vi "count_r3.vi"() -> ()   [LabVIEW 2015]
uses:
  <vilib>/myRIO/Instrument Drivers/Onboard IO/PWM/typedefs/PWM Reference.ctl
  <vilib>/myRIO/Common/Instrument Driver Framework/Utilities/typedefs/myRIO Generic Hardware Reference.ctl
  <vilib>/myRIO/Common/Instrument Driver Framework/Utilities/typedefs/Hardware Version Enum.ctl
  <vilib>/myRIO/Common/Instrument Driver Framework/Utilities/typedefs/myRIO v1.0 Reference.ctl
  <vilib>/myRIO/Common/Instrument Driver Framework/Utilities/typedefs/Generic FPGA Reference.ctl
  <vilib>/myRIO/Common/Instrument Driver Framework/myRIO v1.0/PWM/typedefs/PWM Channels Enum.ctl
  <vilib>/myRIO/Instrument Drivers/Onboard IO/PWM/typedefs/PWM Configuration.ctl
  <vilib>/userdefined/High Color/nirio_resource_hc.ctl
  <vilib>/myRIO/Common/Instrument Driver Framework/myRIO v1.0/PWM/vis/myRIO v1.1 Open PWM.vi
  <vilib>/myRIO/Common/Instrument Driver Framework/Utilities/vis/Validate Channels.vi
  <vilib>/myRIO/Common/Instrument Driver Framework/myRIO v1.0/PWM/vis/myRIO v1.0 Reserve PWM.vi
  <vilib>/myRIO/Instrument Drivers/Onboard IO/PWM/vis/Set Duty Cycle and Frequency.vi
  <vilib>/myRIO/Common/Instrument Driver Framework/myRIO v1.0/PWM/vis/myRIO v1.0 Build MUX Configuration PWM.vi
  <vilib>/myRIO/Common/Instrument Driver Framework/myRIO v1.0/Resource Manager/vis/myRIO v1.0 Reserve Channel List.vi
  <vilib>/myRIO/Common/Instrument Driver Framework/myRIO v1.0/Resource Manager/vis/myRIO v1.0 Create Configuration List.vi
  <vilib>/myRIO/Common/Instrument Driver Framework/myRIO v1.0/Resource Manager/vis/myRIO v1.0 Reserve Channel.vi
  <vilib>/myRIO/Common/Instrument Driver Framework/myRIO v1.0/Resource Manager/vis/myRIO v1.0 Unreserve Channel.vi
  <vilib>/myRIO/Common/Instrument Driver Framework/myRIO v1.0/Resource Manager/vis/myRIO v1.0 Build Mutex Name.vi
  <vilib>/FPGAPlugInAG/myRIO-1900/niLvFpga_Open_myRIO-1900.vi
  <vilib>/rvi/interface/common/dynamic/niFpgaDynamicAddResources.vi
  <vilib>/myRIO/Common/Instrument Driver Framework/Utilities/vis/FPGA Ref Manager.vi
  <vilib>/Utility/error.llb/Error Cluster From Error Code.vi
  <vilib>/myRIO/Common/Instrument Driver Framework/Utilities/vis/Ref Counter.vi
  <vilib>/rvi/errors/niLvFpgaAdjustHostInterfaceError.vi
  <vilib>/Utility/VariantDataType/GetNumericInfo.vi
  <vilib>/myRIO/Common/Instrument Driver Framework/myRIO v1.0/myRIO v1.1 Open.vi
  <vilib>/myRIO/Common/Instrument Driver Framework/Utilities/vis/IO Manager.vi
  <vilib>/myRIO/Common/Instrument Driver Framework/Utilities/vis/Configuration Manager.vi
  <vilib>/myRIO/Common/Instrument Driver Framework/myRIO v1.0/Resource Manager/vis/myRIO v1.0 Configure IO.vi
  <vilib>/myRIO/Common/Instrument Driver Framework/myRIO v1.0/myRIO v1.0 Close.vi
  <vilib>/myRIO/Common/Instrument Driver Framework/myRIO v1.0/PWM/vis/myRIO v1.0 Write PWM.vi
  <vilib>/rvi/interface/nirviOpenFPGA/nirviOpenFPGA.xnode
  FPGA Bitfiles/NavigationProjec_FPGATarget2_FPGAMainNavigati_PWPHW8gwDxI.lvbitx
  <vilib>/rvi/interface/nirviReadWriteControl/nirviReadWriteControl.xnode
  <vilib>/myRIO/Instrument Drivers/Onboard IO/PWM/vis/myRIO PWM Open.xnode
  <vilib>/myRIO/Instrument Drivers/Onboard IO/PWM/PWM.lvlib
  <vilib>/myRIO/Instrument Drivers/Utilities/Utilities.lvlib
  NiFpgaLv.dll
  <vilib>/rvi/interface/Simulation/niFpgaSimulationCallBeginRW.vi
panel:
  in  "graph?":bool
  out "Tick Count(mSec)":u32
  out "reset x y":dbl
  out "XY Graph":cluster{dbl[], dbl[]}(graph)
  out "x traveled":dbl
  out "y traveled":dbl
  out "avg 123":dbl
  out "avg 456":dbl
  out "psi dot":dbl
  out "distance traveled":dbl
  out "y dot":dbl
  out "x dot":dbl
  out "x position":dbl
  out "y position":dbl
  out "X Pos Lin Estimate":dbl
  out "Delta Lin Distance (ft)":dbl
  out "X Position Estimate":dbl
  out "Delta Distance (ft)":dbl
  in  "start y":dbl=3.0
  in  "start x":dbl=1.0
  out "Delta Encoder Array":u32[](array[numeric])
  out "Current Encoder Array":u32[](array[numeric])
  out "Initial Encoder Array":u32[](array[numeric])
  in  "Encoder Reset":bool
  in  "master motor on switch":bool
  out "L Min Linear Velocity (ft/s) 2":dbl
  out "R Min Linear Velocity (ft/s)  2":dbl
  in  "Goal Y":dbl=3.0 format="%#_13g"
  in  "Goal X":dbl=20.0 format="%#_13g"
  out "x+y":dbl
  out "SYS.SELECTA":u8 format="%08b"
  out "ENC.B_c.CNTR":i32
  out "ENC.B_b.CNTR":i32
  out "ENC.B_a.CNTR":i32
  out "ENC.A_c.CNTR":i32
  out "ENC.A_b.CNTR":i32
  out "ENC.A_a.CNTR":i32
  out "Boolean":bool
  in  "R Desired Input Velocity (ft/s) 2":dbl(knob) scale=-4.0..4.0
  in  "front enable":bool
  in  "mid enable":bool
  in  "Rear enable":bool
  in  "Sync L -> R":bool
  in  "R Min Linear Velocity (ft/s)":dbl=-2.0 format="%#_13g"
  in  "R Max Linear Velocity (ft/s)":dbl=2.0 format="%#_13g"
  out "Rotational Velocity (RPS)":dbl
  in  "L Min Linear Velocity (ft/s)":dbl=-2.0 format="%#_13g"
  in  "L Max Linear Velocity (ft/s)":dbl=2.0 format="%#_13g"
  out "Current Rot Velocity (rot/s)":T1(graph)
  in  "L Desired Input Velocity (ft/s)":dbl(knob) scale=-4.0..4.0
  # "Motor Control Parameters"
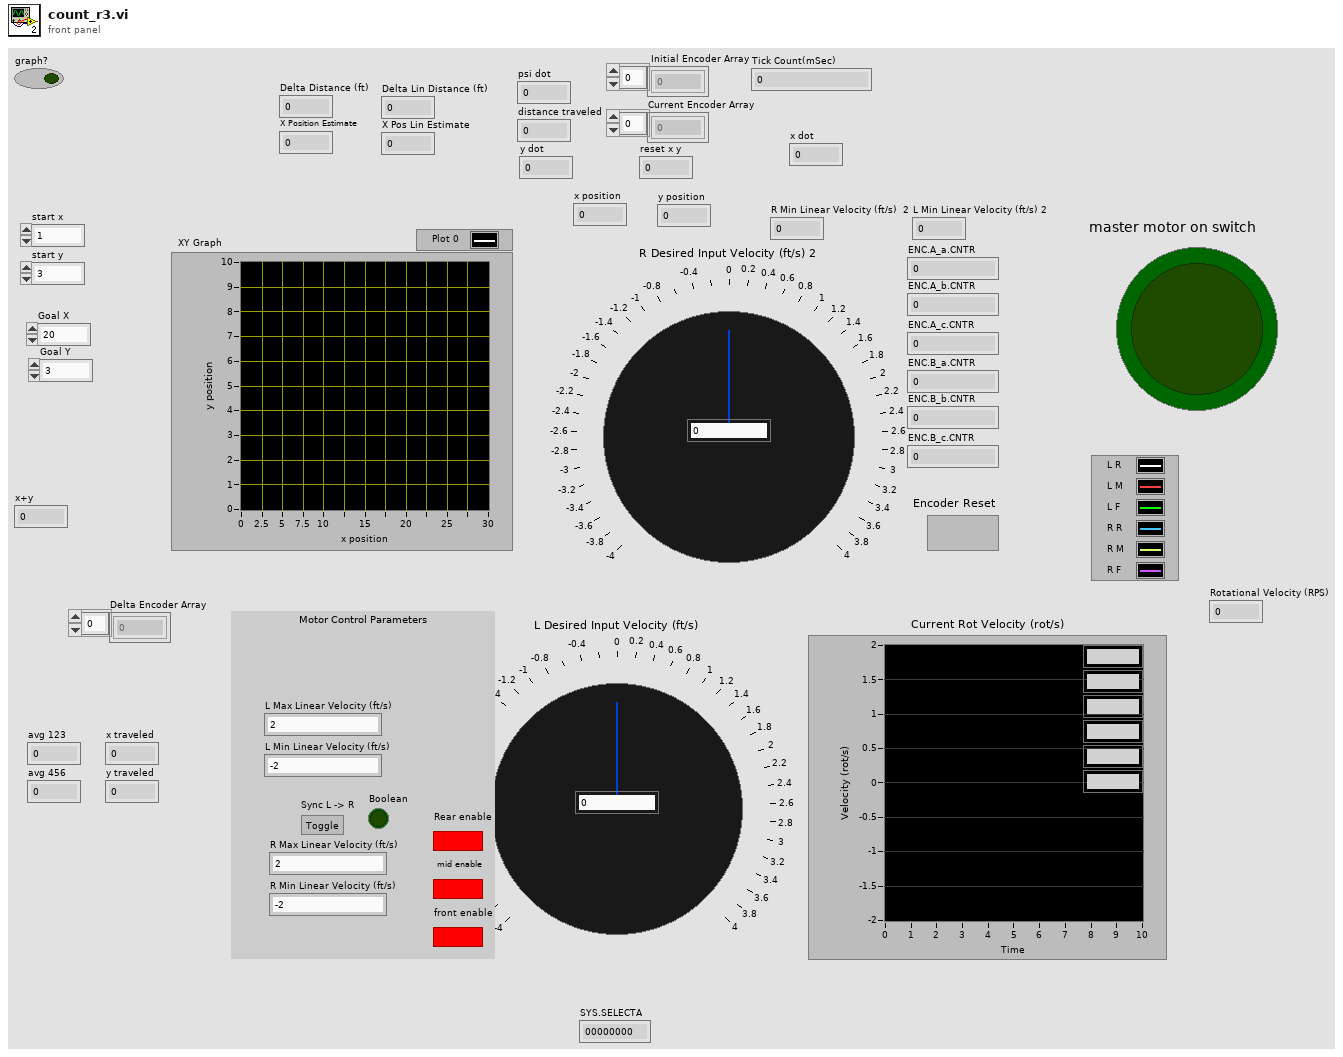
[diagram p1: front panel]
types:
  T1 = cluster{"Rotational Velocity (RPS)":dbl, "Rotational Velocity (RPS)":dbl, "Rotational Velocity (RPS)":dbl, "Rotational Velocity (RPS)":dbl, "Rotational Velocity (RPS)":dbl, "Rotational Velocity (RPS)":dbl}
  T2 = typedef "nirio_resource_hc.ctl" = tag
  T3 = typedef "Hardware Version Enum.ctl" = enum16{"Unknown", "myRIO-1900", "myRIO-1950", "roboRIO"}
  T4 = typedef "PWM.lvlib/PWM Reference.ctl" = cluster{"myRIO Reference":T5, "PWM Channels Enum":T8, "PWM Configuration":T9}
  T5 = typedef "myRIO Generic Hardware Reference.ctl" = cluster{"myRIO Model":T3, "myRIO Hardware Reference":T6}
  T6 = typedef "myRIO v1.0 Reference.ctl" = cluster{"Generic FPGA Reference":T7, "Allow multiple opens":bool}
  T7 = typedef "Generic FPGA Reference.ctl" = refnum<k20>
  T8 = typedef "PWM Channels Enum.ctl" = enum16{"Not Connected", "C/PWM0", "C/PWM1", "A/PWM0", "A/PWM1", "A/PWM2", "B/PWM0", "B/PWM1", "B/PWM2", "PWM/PWM0", "PWM/PWM1", "PWM/PWM2", "PWM/PWM3", "PWM/PWM4", "PWM/PWM5", "PWM/PWM6", "PWM/PWM7", "PWM/PWM8", "PWM/PWM9"}
  T9 = typedef "PWM.lvlib/PWM Configuration.ctl" = cluster{"Frequency":dbl, "Duty Cycle":dbl}
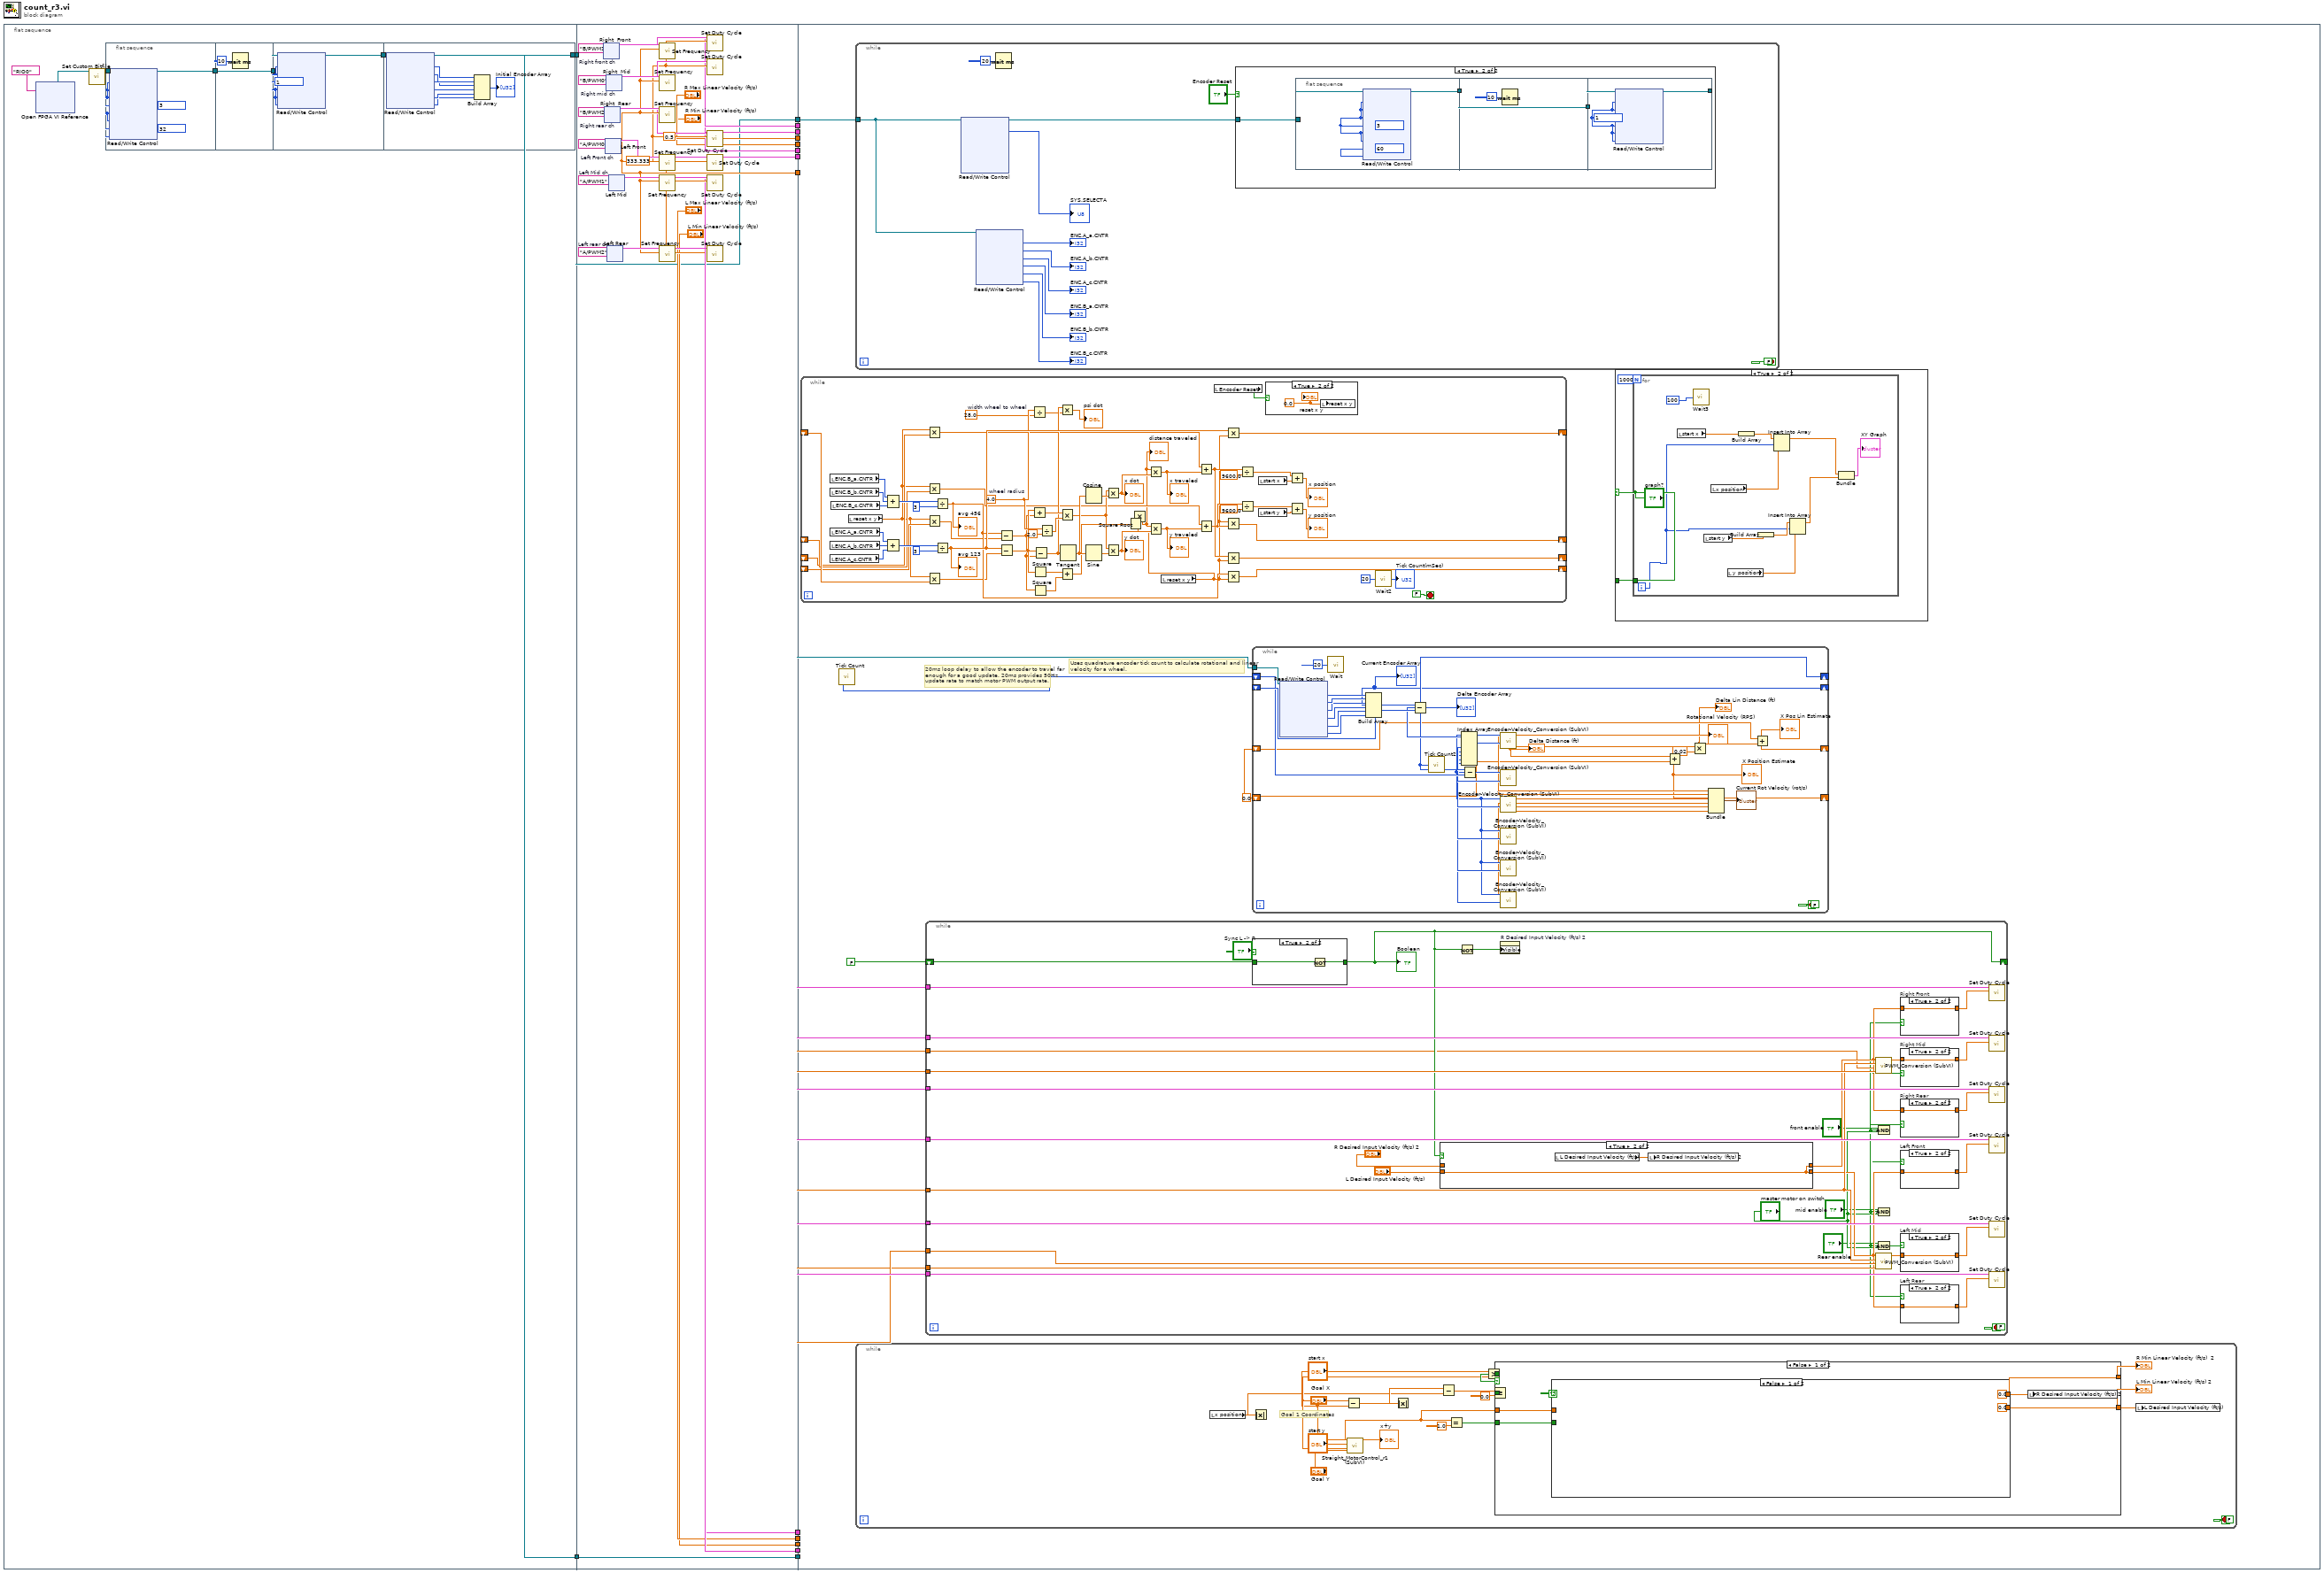
[diagram p0: block diagram]
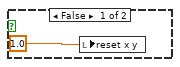
[diagram p3: hidden frame]
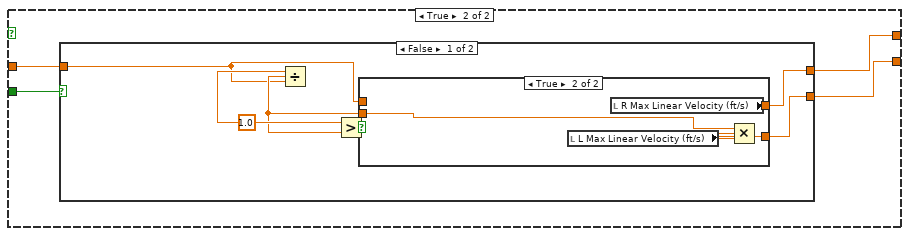
[diagram p4: hidden frame]
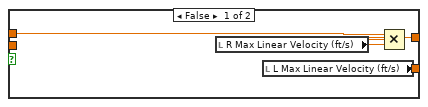
[diagram p5: hidden frame]
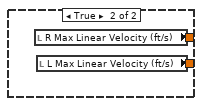
[diagram p6: hidden frame]
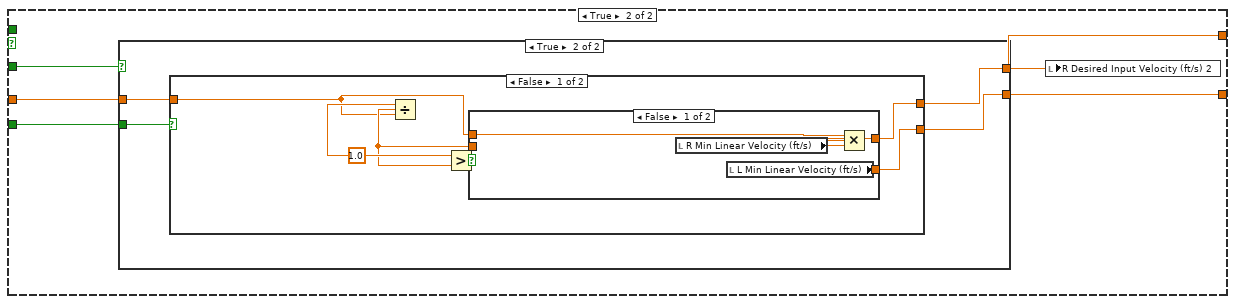
[diagram p7: hidden frame]
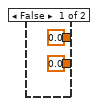
[diagram p8: hidden frame]
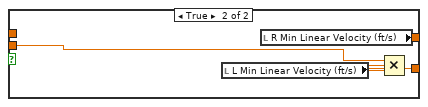
[diagram p9: hidden frame]
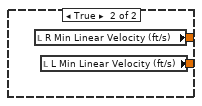
[diagram p10: hidden frame]
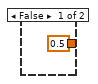
[diagram p13: hidden frame]
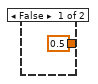
[diagram p14: hidden frame]
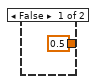
[diagram p15: hidden frame]
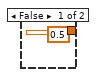
[diagram p16: hidden frame]
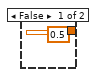
[diagram p17: hidden frame]
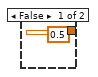
[diagram p18: hidden frame]
diagram:
  n1 = flat-sequence {
    tunnel: [w19] -> w3
    tunnel: [w19] -> w1
    tunnel: [w60] -> w15
    tunnel: [w55] -> w14
    tunnel: [w51] -> w13
    tunnel: [w50] -> w12
    tunnel: [w49] -> w11
    tunnel: [w48] -> w10
    tunnel: [w47] -> w9
    tunnel: ["L Max Linear Velocity (ft/s)"] -> w8
    tunnel: ["L Min Linear Velocity (ft/s)"] -> w7
    tunnel: ["R Max Linear Velocity (ft/s)"] -> w6
    tunnel: ["R Min Linear Velocity (ft/s)"] -> w5
    tunnel: [w42] -> w4
    tunnel: w3 -> [w41]
    tunnel: [w41] -> w2
    tunnel: w1 -> [w42]
    tunnel: w15 -> [w184]
    tunnel: w14 -> [w183]
    tunnel: w13 -> [w182]
    tunnel: w12 -> [w181]
    tunnel: w11 -> [w180]
    tunnel: w10 -> [w179]
    tunnel: w9 -> [w178]
    tunnel: w8 -> [w177]
    tunnel: w7 -> [w176]
    tunnel: w6 -> [w175]
    tunnel: w5 -> [w174]
    tunnel: w4 -> [w172]
    tunnel: w2 -> [w171]
    frame #0 {
      n2 = xnode "Open FPGA VI Reference"("resource name"=tag "RIO0") -> ("FPGA VI Reference Out"=w16:refnum<k20>)  [unwired: 1 in, 1 out]
      n3 = call <vilib>:"Set Custom Bitfile.vi"("Custom FPGA Reference In"=w16) -> ("Custom FPGA Reference Out"=w20:refnum<k20>)  [unwired: 9 in, 1 out]
      n4 = flat-sequence {
        tunnel: w20 -> [w25]
        tunnel: [w23] -> w22
        tunnel: w22 -> [w27]
        tunnel: [w27] -> w21
        tunnel: w21 -> [w30]
        tunnel: [w29] -> w18
        tunnel: [w32] -> w19
        tunnel: w18 -> [w33]
        frame #0 {
          w24 = u8 32 ("SYS.SELECTA")
          w26 = u8 3 ("ENC.B_c.CNFG")
          n5 = xnode "Read/Write Control"("FPGA VI Reference In"=w25, "ENC.A_a.CNFG"=w26, "ENC.A_b.CNFG"=w26, "ENC.A_c.CNFG"=w26, "ENC.B_a.CNFG"=w26, "ENC.B_b.CNFG"=w26, "ENC.B_c.CNFG"=w26, "SYS.SELECTA"=w24, "SYS.SELECTB"=w24) -> ("FPGA VI Reference Out"=w23:refnum<k20>)  [unwired: 1 in, 1 out]
        }
        frame #1 {
          n6 = Wait (ms)(milliseconds to wait=u32 10) -> ()  [unwired: 1 out]
        }
        frame #2 {
          w31 = u8 1 ("ENC.B_c.CNFG")
          n7 = xnode "Read/Write Control"("FPGA VI Reference In"=w30, "ENC.A_a.CNFG"=w31, "ENC.A_b.CNFG"=w31, "ENC.A_c.CNFG"=w31, "ENC.B_a.CNFG"=w31, "ENC.B_b.CNFG"=w31, "ENC.B_c.CNFG"=w31) -> ("FPGA VI Reference Out"=w29:refnum<k20>)  [unwired: 1 in, 1 out]
        }
        frame #3 {
          n8 = xnode "Read/Write Control"("FPGA VI Reference In"=w33) -> ("FPGA VI Reference Out"=w32:refnum<k20>, "ENC.A_a.CNTR"=w40:u32, "ENC.A_b.CNTR"=w39:u32, "ENC.A_c.CNTR"=w38:u32, "ENC.B_a.CNTR"=w37:u32, "ENC.B_b.CNTR"=w36:u32, "ENC.B_c.CNTR"=w35:u32)  [unwired: 1 in, 1 out]
          n9 = Build Array(w40, w39, w38, w37, w36, w35) -> (→"Initial Encoder Array":u32[])
        }
      }
    }
    frame #1 {
      w52 = 0.5 ("Duty Cycle")
      w60 = 333.333 ("Frequency [Hz]")
      w67 = tag "B/PWM2"  # Right rear ch
      w68 = tag "B/PWM0"  # Right mid ch
      w69 = tag "B/PWM1"  # Right front ch
      w70 = tag "A/PWM2"  # Left rear ch
      w71 = tag "A/PWM0"  # Left Front ch
      w72 = tag "A/PWM1"  # Left Mid ch
      n10 = xnode "Right  Front"("Channel Name"=w69) -> ("PWM Ref Out"=w63:T4)  [unwired: 2 in, 1 out]
      n11 = xnode "Right  Rear"("Channel Name"=w67) -> ("PWM Ref Out"=w61:T4)  [unwired: 2 in, 1 out]
      n12 = xnode "Left Front"("Channel Name"=w71) -> ("PWM Ref Out"=w65:T4)  [unwired: 2 in, 1 out]
      n13 = xnode "Right  Mid"("Channel Name"=w68) -> ("PWM Ref Out"=w62:T4)  [unwired: 2 in, 1 out]
      n14 = xnode "Left Rear"("Channel Name"=w70) -> ("PWM Ref Out"=w64:T4)  [unwired: 2 in, 1 out]
      n15 = xnode "Left Mid"("Channel Name"=w72) -> ("PWM Ref Out"=w66:T4)  [unwired: 2 in, 1 out]
      n16 = call <vilib>:"Set Frequency.vi"("Frequency [Hz]"=w60, "PWM Ref In"=w63) -> ("PWM Ref Out"=w56:T4)  [unwired: 7 in, 1 out]
      n17 = call <vilib>:"Set Frequency.vi"("Frequency [Hz]"=w60, "PWM Ref In"=w62) -> ("PWM Ref Out"=w57:T4)  [unwired: 7 in, 1 out]
      n18 = call <vilib>:"Set Frequency.vi"("Frequency [Hz]"=w60, "PWM Ref In"=w61) -> ("PWM Ref Out"=w58:T4)  [unwired: 7 in, 1 out]
      n19 = call <vilib>:"Set Frequency.vi"("Frequency [Hz]"=w60, "PWM Ref In"=w65) -> ("PWM Ref Out"=w53:T4)  [unwired: 7 in, 1 out]
      n20 = call <vilib>:"Set Frequency.vi"("Frequency [Hz]"=w60, "PWM Ref In"=w66) -> ("PWM Ref Out"=w59:T4)  [unwired: 7 in, 1 out]
      n21 = call <vilib>:"Set Frequency.vi"("Frequency [Hz]"=w60, "PWM Ref In"=w64) -> ("PWM Ref Out"=w54:T4)  [unwired: 7 in, 1 out]
      n22 = call <vilib>:"Set Duty Cycle.vi"("Duty Cycle"=w52, "PWM Ref In"=w56) -> ("PWM Ref Out"=w51:T4)  [unwired: 7 in, 1 out]
      n23 = call <vilib>:"Set Duty Cycle.vi"("Duty Cycle"=w52, "PWM Ref In"=w57) -> ("PWM Ref Out"=w50:T4)  [unwired: 7 in, 1 out]
      n24 = call <vilib>:"Set Duty Cycle.vi"("Duty Cycle"=w52, "PWM Ref In"=w58) -> ("PWM Ref Out"=w49:T4)  [unwired: 7 in, 1 out]
      n25 = call <vilib>:"Set Duty Cycle.vi"("Duty Cycle"=w52, "PWM Ref In"=w53) -> ("PWM Ref Out"=w48:T4)  [unwired: 7 in, 1 out]
      n26 = call <vilib>:"Set Duty Cycle.vi"("Duty Cycle"=w52, "PWM Ref In"=w59) -> ("PWM Ref Out"=w47:T4)  [unwired: 7 in, 1 out]
      n27 = call <vilib>:"Set Duty Cycle.vi"("Duty Cycle"=w52, "PWM Ref In"=w54) -> ("PWM Ref Out"=w55:T4)  [unwired: 7 in, 1 out]
    }
    frame #2 {
      w170 = 0.0
      # "Uses quadrature encoder tick count to calculate rotational and linear velocity for a wheel."
      # "20ms loop delay to allow the encoder to travel far enough for a good update. 20ms provides 50Hz update rate to match motor PWM output rate."
      n28 = while {
        shift-right: [w209] -> _
        shift-left: _ -> [w248]
        shift-right: [w206] -> _
        shift-left: _ -> [w247]
        shift-right: [w208] -> _
        shift-left: _ -> [w221]
        shift-right: [w207] -> _
        shift-left: _ -> [w220]
        stop <- FALSE stop-if-true
        w243 = 28.0  # width wheel to wheel
        w244 = 4.0  # wheel radius
        n29 = local read "ENC.B_a.CNTR"() -> (w253:i32)
        n30 = local read "ENC.B_b.CNTR"() -> (w252:i32)
        n31 = local read "ENC.A_a.CNTR"() -> (w256:i32)
        n32 = local read "ENC.A_b.CNTR"() -> (w255:i32)
        n33 = local read "ENC.A_c.CNTR"() -> (w254:i32)
        n34 = local read "ENC.B_c.CNTR"() -> (w251:i32)
        n35 = local read "reset x y"() -> (w205:dbl)
        n36 = Compound Arithmetic op=ADD(w253, w252, w251) -> (w259:i32)
        n37 = Compound Arithmetic op=ADD(w256, w255, w254) -> (w260:i32)
        n38 = Multiply(x=w205, y=w220) -> (x*y=w211:dbl)
        n39 = Multiply(x=w205, y=w221) -> (x*y=w212:dbl)
        n40 = Multiply(x=w205, y=w247) -> (x*y=w210:dbl)
        n41 = Multiply(x=w205, y=w248) -> (x*y=w213:dbl)
        n42 = Divide(x=w259, y=3) -> (x/y=w246:dbl)
        "avg 456" <- w246
        n43 = Divide(x=w260, y=3) -> (x/y=w249:dbl)
        "avg 123" <- w249
        n44 = Subtract(x=w246, y=w210) -> (x-y=w235:dbl)
        n45 = Subtract(x=w249, y=w213) -> (x-y=w236:dbl)
        n46 = Divide(x=w244, y=w243) -> (x/y=w239:dbl)
        n47 = Add(x=w236, y=w235) -> (x+y=w241:dbl)
        n48 = Square(x=w236) -> (x^2=w233:dbl)
        n49 = Square(x=w235) -> (x^2=w234:dbl)
        n50 = Subtract(x=w236, y=w235) -> (x-y=w240:dbl)
        n51 = Divide(x=w244, y=2.0) -> (x/y=w242:dbl)
        n52 = Multiply(x=w240, y=w239) -> (x*y=→"psi dot":dbl)
        n53 = Multiply(x=w241, y=w242) -> (x*y=w229:dbl)
        n54 = Add(x=w233, y=w234) -> (x+y=w232:dbl)
        n55 = Tangent(1:w240) -> (0:w237:dbl)
        n56 = Cosine(x=w237) -> (cos(x)=w230:dbl)
        n57 = Sine(x=w237) -> (sin(x)=w231:dbl)
        n58 = Multiply(x=w229, y=w230) -> (x*y=w227:dbl)
        "x dot" <- w227
        n59 = Multiply(x=w229, y=w231) -> (x*y=w228:dbl)
        "y dot" <- w228
        n60 = Square Root(x=w232) -> (sqrt(x)=w226:dbl)
        n61 = local read "reset x y"() -> (w203:dbl)
        n62 = Multiply(x=w226, y=w203) -> (x*y=w204:dbl)
        "distance traveled" <- w204
        n63 = Multiply(x=w204, y=w227) -> (x*y=w225:dbl)
        "x traveled" <- w225
        n64 = Multiply(x=w204, y=w228) -> (x*y=w224:dbl)
        "y traveled" <- w224
        n65 = Add(x=w211, y=w225) -> (x+y=w223:dbl)
        n66 = Add(x=w212, y=w224) -> (x+y=w215:dbl)
        n67 = local read "Encoder Reset"() -> (w202:bool)
        n68 = Multiply(x=w249, y=w203) -> (x*y=w209:dbl)
        n69 = Multiply(x=w203, y=w215) -> (x*y=w208:dbl)
        n70 = Multiply(x=w223, y=w203) -> (x*y=w207:dbl)
        n71 = Multiply(x=w246, y=w203) -> (x*y=w206:dbl)
        n72 = Divide(x=w223, y=9600.0) -> (x/y=w218:dbl)
        n73 = Divide(x=w215, y=9600.0) -> (x/y=w219:dbl)
        n74 = local read "start x"() -> (w216:dbl)
        n75 = local read "start y"() -> (w217:dbl)
        n76 = case shown="True" w202 {
          frame False {
            n77 = local write "reset x y"(1.0) -> ()
          }
          frame True {
            w263 = 0.0
            n78 = local write "reset x y"(w263) -> ()
            "reset x y" <- w263
          }
        }
        n79 = Add(x=w218, y=w216) -> (x+y=→"x position":dbl)
        n80 = Add(x=w219, y=w217) -> (x+y=→"y position":dbl)
        n81 = call "Wait2"("Count(mSec)"=u32 20) -> ("Tick Count(mSec)"=→"Tick Count(mSec)":u32)
      }
      n82 = call "Tick Count"() -> ("Tick Count(uSec)"=w185:u32)
      n83 = while {
        tunnel: w172 -> [w339]
        stop <- FALSE stop-if-true
        n84 = xnode "Read/Write Control"("FPGA VI Reference In"=w339) -> ("FPGA VI Reference Out"=w337:refnum<k20>, "SYS.SELECTA"=→"SYS.SELECTA":u8)  [unwired: 1 in, 6 out]
        n85 = xnode "Read/Write Control"("FPGA VI Reference In"=w339) -> ("ENC.A_a.CNTR"=→"ENC.A_a.CNTR":u32, "ENC.A_b.CNTR"=→"ENC.A_b.CNTR":u32, "ENC.A_c.CNTR"=→"ENC.A_c.CNTR":u32, "ENC.B_a.CNTR"=→"ENC.B_a.CNTR":u32, "ENC.B_b.CNTR"=→"ENC.B_b.CNTR":u32, "ENC.B_c.CNTR"=→"ENC.B_c.CNTR":u32)  [unwired: 1 in, 2 out]
        n86 = Wait (ms)(milliseconds to wait=u32 20) -> ()  [unwired: 1 out]
        n87 = case shown="True" "Encoder Reset" {
          tunnel: w337 -> [_ w348]
          frame False {
          }
          frame True {
            n88 = flat-sequence {
              tunnel: w348 -> [w353]
              tunnel: [w351] -> w350
              tunnel: w350 -> [w355]
              tunnel: [w355] -> w349
              tunnel: w349 -> [w358]
              tunnel: [w357] -> _
              frame #0 {
                w352 = u8 60 ("SYS.SELECTA")
                w354 = u8 3 ("ENC.B_c.CNFG")
                n89 = xnode "Read/Write Control"("FPGA VI Reference In"=w353, "ENC.A_a.CNFG"=w354, "ENC.A_b.CNFG"=w354, "ENC.A_c.CNFG"=w354, "ENC.B_a.CNFG"=w354, "ENC.B_b.CNFG"=w354, "ENC.B_c.CNFG"=w354, "SYS.SELECTA"=w352, "SYS.SELECTB"=w352) -> ("FPGA VI Reference Out"=w351:refnum<k20>)  [unwired: 1 in, 1 out]
              }
              frame #1 {
                n90 = Wait (ms)(milliseconds to wait=u32 10) -> ()  [unwired: 1 out]
              }
              frame #2 {
                w359 = u8 1 ("ENC.B_c.CNFG")
                n91 = xnode "Read/Write Control"("FPGA VI Reference In"=w358, "ENC.A_a.CNFG"=w359, "ENC.A_b.CNFG"=w359, "ENC.A_c.CNFG"=w359, "ENC.B_a.CNFG"=w359, "ENC.B_b.CNFG"=w359, "ENC.B_c.CNFG"=w359) -> ("FPGA VI Reference Out"=w357:refnum<k20>)  [unwired: 1 in, 1 out]
              }
            }
          }
        }
      }
      n92 = while {
        stop <- FALSE stop-if-true
        # "Goal 1 Coordinates"
        n93 = local read "x position"() -> (w271:dbl)
        n94 = Absolute Value(x=w271) -> (abs(x)=w265:dbl)
        n95 = Subtract(x="Goal X", y="start x") -> (x-y=w267:dbl)
        n96 = call "Straight_MotorControl_r1 (SubVI).vi"("Goal Y Coord"="Goal Y", "Goal X Coord"="Goal X", "Current Y Pos"="start y", "Current X Pos"="start x") -> ("Numeric Out Y"=w281:dbl)  [unwired: 7 in]
        "x+y" <- w281
        n97 = Absolute Value(x=w267) -> (abs(x)=w266:dbl)
        n98 = Subtract(x=w266, y=w265) -> (x-y=w264:dbl)
        n99 = Equal?(x=w281, y=1.0) -> (x = y?=w279:bool)
        n100 = Greater?(x="start x", y="Goal X") -> (0:w270:bool)
        n101 = Greater Or Equal?(x=w264, y=0.0) -> (x >= y?=w272:bool)
        n102 = case shown="False" w270 {
          tunnel: w281 -> [w284 w313]
          tunnel: w279 -> [w283 w312]
          tunnel: [w286 w311] -> w277
          tunnel: [w285 w310] -> w276
          tunnel: w272 -> [_ w309]
          tunnel: w270 -> [_ _]
          frame False {
            n103 = case shown="False" TRUE {
              tunnel: w284 -> [_ w292]
              tunnel: w283 -> [_ w291]
              tunnel: [0.0 ("R Min Linear Velocity (ft/s)") w290] -> w286
              tunnel: [0.0 ("L Min Linear Velocity (ft/s)") w289] -> w285
              frame False {
              }
              frame True {
                n104 = case shown="False" w291 {
                  tunnel: [w295 w307] -> w289
                  tunnel: [w294 w308] -> w290
                  tunnel: w292 -> [w293 _]
                  frame False {
                    w298 = 1.0 ("x")
                    n105 = Divide(x=w298, y=w293) -> (x/y=w297:dbl)
                    n106 = Greater?(x=w298, y=w297) -> (0:w296:bool)
                    n107 = case shown="True" w296 {
                      tunnel: w297 -> [_ w306]
                      tunnel: [w299 w304] -> w295
                      tunnel: [w300 w303] -> w294
                      tunnel: w293 -> [w302 _]
                      frame False {
                        n108 = local read "R Max Linear Velocity (ft/s)"() -> (w301:dbl)
                        n109 = local read "L Max Linear Velocity (ft/s)"() -> (w299:dbl)
                        n110 = Multiply(x=w302, y=w301) -> (x*y=w300:dbl)
                      }
                      frame True {
                        n111 = local read "L Max Linear Velocity (ft/s)"() -> (w305:dbl)
                        n112 = local read "R Max Linear Velocity (ft/s)"() -> (w303:dbl)
                        n113 = Multiply(x=w306, y=w305) -> (x*y=w304:dbl)
                      }
                    }
                  }
                  frame True {
                    n114 = local read "R Max Linear Velocity (ft/s)"() -> (w308:dbl)
                    n115 = local read "L Max Linear Velocity (ft/s)"() -> (w307:dbl)
                  }
                }
              }
            }
            n116 = local write "R Desired Input Velocity (ft/s) 2"(w286) -> ()
          }
          frame True {
            n117 = case shown="True" w309 {
              tunnel: w313 -> [_ w319]
              tunnel: w312 -> [_ w318]
              tunnel: [0.0 ("R Min Linear Velocity (ft/s)") w317] -> w311
              tunnel: [0.0 ("L Min Linear Velocity (ft/s)") w316] -> w310
              frame False {
              }
              frame True {
                n118 = case shown="False" w318 {
                  tunnel: [w322 w334] -> w316
                  tunnel: [w321 w335] -> w317
                  tunnel: w319 -> [w320 _]
                  frame False {
                    w325 = 1.0 ("x")
                    n119 = Divide(x=w325, y=w320) -> (x/y=w324:dbl)
                    n120 = Greater?(x=w325, y=w324) -> (0:w323:bool)
                    n121 = case shown="False" w323 {
                      tunnel: w324 -> [_ w333]
                      tunnel: [w326 w331] -> w322
                      tunnel: [w327 w330] -> w321
                      tunnel: w320 -> [w329 _]
                      frame False {
                        n122 = local read "R Min Linear Velocity (ft/s)"() -> (w328:dbl)
                        n123 = local read "L Min Linear Velocity (ft/s)"() -> (w326:dbl)
                        n124 = Multiply(x=w329, y=w328) -> (x*y=w327:dbl)
                      }
                      frame True {
                        n125 = local read "L Min Linear Velocity (ft/s)"() -> (w332:dbl)
                        n126 = local read "R Min Linear Velocity (ft/s)"() -> (w330:dbl)
                        n127 = Multiply(x=w333, y=w332) -> (x*y=w331:dbl)
                      }
                    }
                  }
                  frame True {
                    n128 = local read "R Min Linear Velocity (ft/s)"() -> (w335:dbl)
                    n129 = local read "L Min Linear Velocity (ft/s)"() -> (w334:dbl)
                  }
                }
              }
            }
            n130 = local write "R Desired Input Velocity (ft/s) 2"(w311) -> ()
          }
        }
        "R Min Linear Velocity (ft/s)  2" <- w277
        "L Min Linear Velocity (ft/s) 2" <- w276
        n131 = local write "L Desired Input Velocity (ft/s)"(w276) -> ()
      }
      n132 = while {
        tunnel: w184 -> [w378]
        tunnel: w183 -> [w388]
        tunnel: w182 -> [w393]
        tunnel: w181 -> [w392]
        tunnel: w180 -> [w391]
        tunnel: w179 -> [w390]
        tunnel: w178 -> [w389]
        tunnel: w177 -> [w381]
        tunnel: w176 -> [w380]
        tunnel: w175 -> [w367]
        tunnel: w174 -> [w379]
        shift-right: [w368] -> _
        shift-left: FALSE -> [w369]
        stop <- FALSE stop-if-true
        n133 = case shown="True" "Sync L -> R" {
          tunnel: w369 -> [w395 w397]
          tunnel: [w395 w396] -> w368
          frame False {
          }
          frame True {
            n134 = Not(x=w397) -> (.not. x?=w396:bool)
          }
        }
        "Boolean" <- w368
        n135 = case shown="True" w368 {
          tunnel: "L Desired Input Velocity (ft/s)" -> [w411 w412]
          tunnel: [w411 w412] -> w374
          tunnel: "R Desired Input Velocity (ft/s) 2" -> [w410 _]
          tunnel: [w410 w412] -> w372
          frame False {
          }
          frame True {
            n136 = local read "L Desired Input Velocity (ft/s)"() -> (w413:dbl)
            n137 = local write "R Desired Input Velocity (ft/s) 2"(w413) -> ()
          }
        }
        n138 = Not(x=w368) -> (.not. x?=w371:bool)
        n139 = property on="R Desired Input Velocity (ft/s) 2" class="Knob (strict)"("Visible"=w371) -> ()  [unwired: 2 in, 2 out]
        n140 = call "PWM_Conversion (SubVI).vi"("Min Linear Velocity (ft/s)"=w379, "Max Linear Velocity (ft/s)"=w367, "PWM Frequency"=w378, "Linear Velocity Input (ft/s)"=w372) -> ("PWM Signal Output"=w376:dbl)  [unwired: 7 in]
        n141 = call "PWM_Conversion (SubVI).vi"("Min Linear Velocity (ft/s)"=w380, "Max Linear Velocity (ft/s)"=w381, "PWM Frequency"=w378, "Linear Velocity Input (ft/s)"=w374) -> ("PWM Signal Output"=w377:dbl)  [unwired: 7 in]
        n142 = Compound Arithmetic op=AND("front enable", "master motor on switch") -> (w361:bool)
        n143 = Compound Arithmetic op=AND("mid enable", "master motor on switch") -> (w360:bool)
        n144 = Compound Arithmetic op=AND("Rear enable", "master motor on switch") -> (w362:bool)
        n145 = case "Right Front" shown="True" w361 {
          tunnel: [0.5 w409] -> w382
          tunnel: w376 -> [_ w409]
          frame False {
          }
          frame True {
          }
        }
        n146 = case "Right Mid" shown="True" w360 {
          tunnel: [0.5 w407] -> w383
          tunnel: w376 -> [_ w407]
          frame False {
          }
          frame True {
          }
        }
        n147 = case "Right Rear" shown="True" w362 {
          tunnel: [0.5 w405] -> w384
          tunnel: w376 -> [_ w405]
          frame False {
          }
          frame True {
          }
        }
        n148 = case "Left Front" shown="True" w361 {
          tunnel: [0.5 w403] -> w385
          tunnel: w377 -> [_ w403]
          frame False {
          }
          frame True {
          }
        }
        n149 = case "Left Mid" shown="True" w360 {
          tunnel: [0.5 w401] -> w386
          tunnel: w377 -> [_ w401]
          frame False {
          }
          frame True {
          }
        }
        n150 = case "Left Rear" shown="True" w362 {
          tunnel: [0.5 w399] -> w387
          tunnel: w377 -> [_ w399]
          frame False {
          }
          frame True {
          }
        }
        n151 = call <vilib>:"Set Duty Cycle.vi"("Duty Cycle"=w382, "PWM Ref In"=w393) -> ()  [unwired: 7 in, 2 out]
        n152 = call <vilib>:"Set Duty Cycle.vi"("Duty Cycle"=w383, "PWM Ref In"=w392) -> ()  [unwired: 7 in, 2 out]
        n153 = call <vilib>:"Set Duty Cycle.vi"("Duty Cycle"=w384, "PWM Ref In"=w391) -> ()  [unwired: 7 in, 2 out]
        n154 = call <vilib>:"Set Duty Cycle.vi"("Duty Cycle"=w385, "PWM Ref In"=w390) -> ()  [unwired: 7 in, 2 out]
        n155 = call <vilib>:"Set Duty Cycle.vi"("Duty Cycle"=w386, "PWM Ref In"=w389) -> ()  [unwired: 7 in, 2 out]
        n156 = call <vilib>:"Set Duty Cycle.vi"("Duty Cycle"=w387, "PWM Ref In"=w388) -> ()  [unwired: 7 in, 2 out]
      }
      n157 = while {
        shift-right: [w422] -> _
        shift-left: _ -> [w440]
        shift-right: [w438] -> _
        shift-left: w185 -> [w437]
        tunnel: w171 -> [w447]
        shift-right: [w419] -> _
        shift-left: w170 -> [w420]
        shift-right: [w414] -> _
        shift-left: w170 -> [w416]
        stop <- FALSE stop-if-true
        n158 = xnode "Read/Write Control"("FPGA VI Reference In"=w447) -> ("ENC.A_a.CNTR"=w446:u32, "ENC.A_b.CNTR"=w445:u32, "ENC.A_c.CNTR"=w444:u32, "ENC.B_a.CNTR"=w443:u32, "ENC.B_b.CNTR"=w442:u32, "ENC.B_c.CNTR"=w441:u32)  [unwired: 1 in, 2 out]
        n159 = call "Wait"("Count(mSec)"=u32 20) -> ()  [unwired: 1 out]
        n160 = Build Array(w446, w445, w444, w443, w442, w441) -> (w422:u32[])
        "Current Encoder Array" <- w422
        n161 = Subtract(x=w422, y=w440) -> (x-y=w439:u32[])
        "Delta Encoder Array" <- w439
        n162 = call "Tick Count2"() -> ("Tick Count(uSec)"=w438:u32)
        n163 = Index Array(array=w439) -> (element #1=w436:u32, element #2=w435:u32, element #3=w434:u32, element #4=w433:u32, element #5=w432:u32, element #6=w431:u32)  [unwired: 6 in]
        n164 = Subtract(x=w438, y=w437) -> (x-y=w430:u32)
        n165 = call "Encoder-Velocity_Conversion (SubVI).vi"("delta  Encoder Count"=w436, "dt (uSec)"=w430) -> ("Distance (ft)"=w421:dbl, "Linear Velocity (ft/s)"=w418:dbl, "Rotational Velocity (RPS)"=w429:dbl)  [unwired: 7 in]
        "Rotational Velocity (RPS)" <- w429
        "Delta Distance (ft)" <- w421
        n166 = call "Encoder-Velocity_Conversion (SubVI).vi"("delta  Encoder Count"=w435, "dt (uSec)"=w430) -> ("Rotational Velocity (RPS)"=w428:dbl)  [unwired: 7 in, 2 out]
        n167 = call "Encoder-Velocity_Conversion (SubVI).vi"("delta  Encoder Count"=w434, "dt (uSec)"=w430) -> ("Rotational Velocity (RPS)"=w427:dbl)  [unwired: 7 in, 2 out]
        n168 = call "Encoder-Velocity_Conversion (SubVI).vi"("delta  Encoder Count"=w433, "dt (uSec)"=w430) -> ("Rotational Velocity (RPS)"=w426:dbl)  [unwired: 7 in, 2 out]
        n169 = call "Encoder-Velocity_Conversion (SubVI).vi"("delta  Encoder Count"=w432, "dt (uSec)"=w430) -> ("Rotational Velocity (RPS)"=w425:dbl)  [unwired: 7 in, 2 out]
        n170 = call "Encoder-Velocity_Conversion (SubVI).vi"("delta  Encoder Count"=w431, "dt (uSec)"=w430) -> ("Rotational Velocity (RPS)"=w424:dbl)  [unwired: 7 in, 2 out]
        n171 = Add(x=w421, y=w420) -> (x+y=w419:dbl)
        "X Position Estimate" <- w419
        n172 = Multiply(x=w418, y=0.02) -> (x*y=w415:dbl)
        "Delta Lin Distance (ft)" <- w415
        n173 = Bundle("Rotational Velocity (RPS)"=w429, "Rotational Velocity (RPS)"=w428, "Rotational Velocity (RPS)"=w427, "Rotational Velocity (RPS)"=w426, "Rotational Velocity (RPS)"=w425, "Rotational Velocity (RPS)"=w424) -> (→"Current Rot Velocity (rot/s)":T1)  [unwired: 1 in]
        n174 = Add(x=w416, y=w415) -> (x+y=w414:dbl)
        "X Pos Lin Estimate" <- w414
      }
      n175 = case shown="True" "graph?" {
        tunnel: "graph?" -> [_ w187]
        frame False {
        }
        frame True {
          n176 = for {
            N: 1000 -> [_]
            tunnel: w187 -> [_]
            i -> [w189]
            n177 = local read "start x"() -> (w197:dbl)
            n178 = call "Wait3"("Count(mSec)"=u32 100) -> ()  [unwired: 1 out]
            n179 = local read "start y"() -> (w192:dbl)
            n180 = local read "x position"() -> (w195:dbl)
            n181 = local read "y position"() -> (w194:dbl)
            n182 = Build Array(w197) -> (w196:dbl[])
            n183 = Build Array(w192) -> (w193:dbl[])
            n184 = Insert Into Array(array=w196, index=w189, new element=w195) -> (w191:dbl[])
            n185 = Insert Into Array(array=w193, index=w189, new element=w194) -> (w190:dbl[])
            n186 = Bundle(w191, w190) -> (→"XY Graph":cluster{dbl[], dbl[]})  [unwired: 1 in]
          }
        }
      }
    }
  }
